vi "UserInput-Button.vi"() -> ()   [LabVIEW 2019]
panel:
  in  "Push Button Control":bool
  out "Round LED":bool
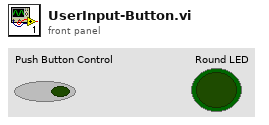
[diagram p1: front panel]
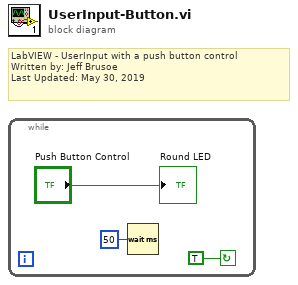
[diagram p0: block diagram]
diagram:
  # "LabVIEW - UserInput with a push button control\nWritten by: Jeff Brusoe\nLast Updated: May 30, 2019"
  n1 = while {
    stop <- TRUE continue-if-true
    n2 = Wait (ms)(milliseconds to wait=u32 50) -> ()  [unwired: 1 out]
    "Round LED" <- "Push Button Control"
  }
